vi "Cleanup Minesweeper Drawing Event.vi"(8 "Error In":errorcluster, 10 "user event":refnum<user-event>, 11 "Event Registration Refnum":refnum<event-registration>) -> (0 "Error Out":errorcluster)   [LabVIEW 2011]
uses:
  Minesweeper Drawing Event Type Def.ctl
  Minesweeper Drawing Operation Type Def.ctl
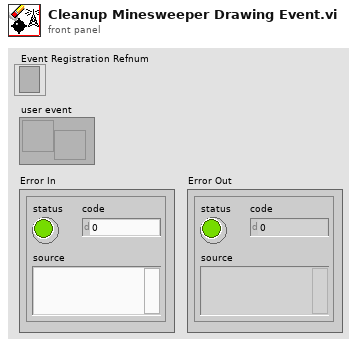
[diagram p1: front panel]
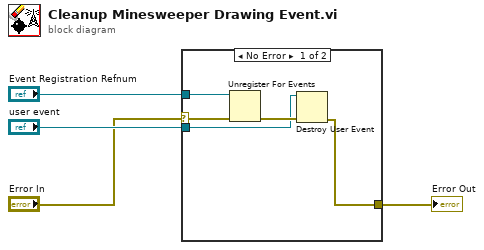
[diagram p0: block diagram]
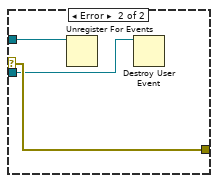
[diagram p2: hidden frame]
diagram:
  n1 = case shown="No Error" "Error In" {
    selector: "Error In" -> [w5 w12]
    tunnel: "Event Registration Refnum" -> [w8 w11]
    tunnel: "user event" -> [w7 w10]
    tunnel: [w6 w12] -> w2
    frame No Error {
      n2 = Unregister For Events(event registration refnum=w8, error in=w5) -> (error out=w9:errorcluster)
      n3 = Destroy User Event(user event=w7, error in=w9) -> (error out=w6:errorcluster)
    }
    frame Error {
      n4 = Unregister For Events(event registration refnum=w11) -> ()  [unwired: 1 in, 1 out]
      n5 = Destroy User Event(user event=w10) -> ()  [unwired: 1 in, 1 out]
    }
  }
  "Error Out" <- w2
